vi "get_ValuesByKeyString.vi"(10 "keyString":string, 11 "Json Input":string="{\"code\": 111, \"msg\": \"success\", \"data\": {\"camera_udp_port\": 10001, \"radar_udp_port\": 17000, \"radar_decode_head\": \"AAAA5555\", \"tcp_server_port\": 8888, \"mcu_enable\": 1, \"ntp_enable\": 1, \"radar_get_edition_enable\": 1, \"mcu_get_edition_enable\": 1, \"infer_enable\": 1, \"cpu_min_to_restart_infer\": 20, \"camera_remote_enable\": 1, \"video_save\": 3, \"pronounce_english\": 0, \"zipx_s_service_restart_time_s\": -1, \"http_file_port\": -1, \"max_file_num\": 1000, \"max_file_size\": 2000000000, \"pic_timeSpan_min\": 5, \"mp4_timeSpan_min\": 4, \"pika_rabbitmq_enable\": 0, \"pika_sftp_enable\": 0, \"radar_alarm_score\": 455, \"camera_alarm_score\": 20, \"joint_alarm_score\": 150, \"camera_radar_h_offset_rad\": -0.01, \"confidence_min\": 0.55, \"radarOffset\": 0.0, \"autoMendRadarOffset\": 0, \"autoCalibration\": 0, \"H\": 2.4}}") -> (3 "Values":dbl[](array[numeric]))   [LabVIEW 2022 SP3]
uses:
  <vilib>/Utility/error.llb/Trim Whitespace One-Sided.vi
panel:
  out "Array":string[](array[string])
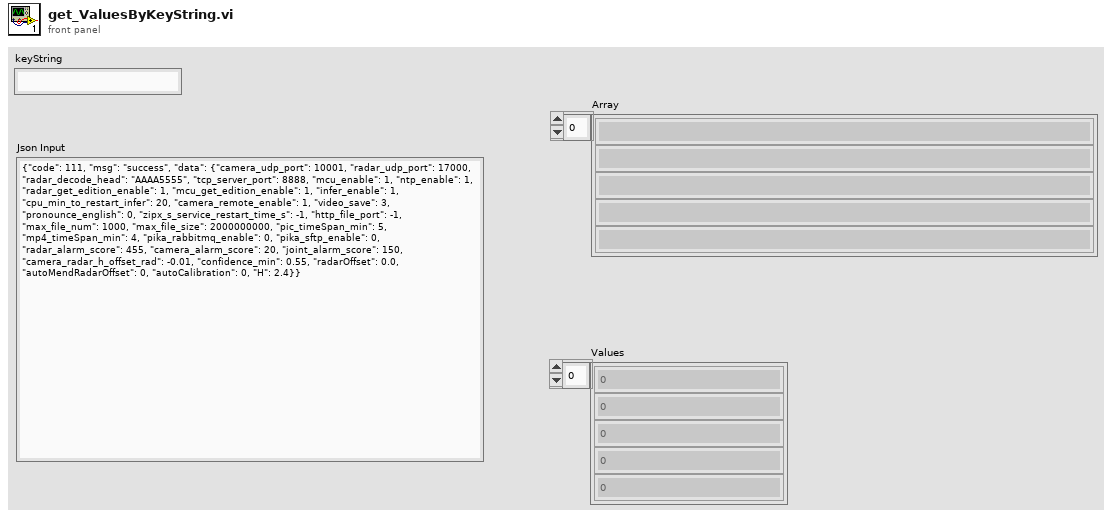
[diagram p1: front panel]
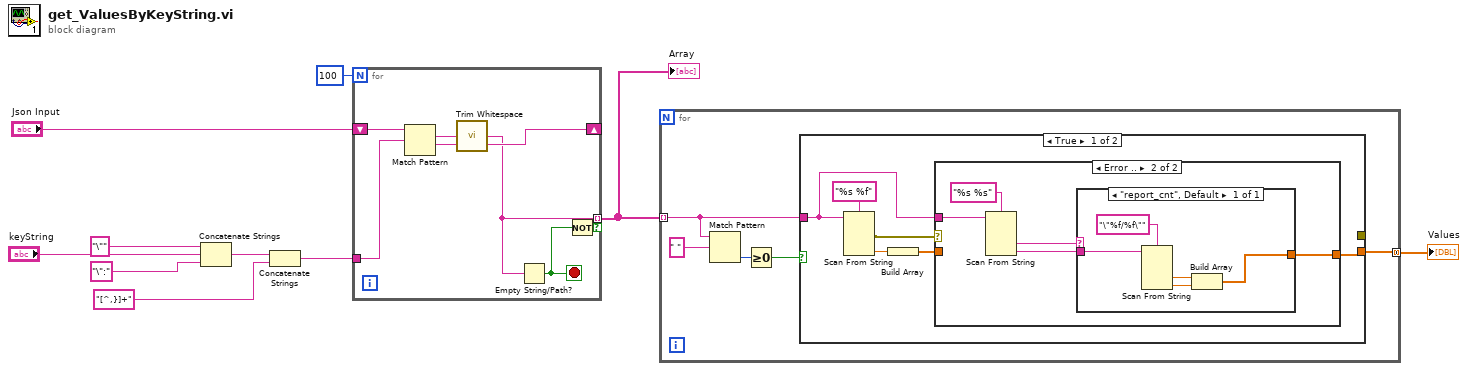
[diagram p0: block diagram]
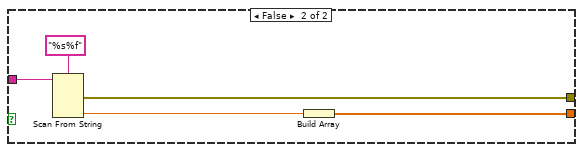
[diagram p3: hidden frame]
diagram:
  n1 = Concatenate Strings("\"" ("string"), "keyString", "\":" ("regular expression")) -> (w6:string)
  n2 = Concatenate Strings(w6, "[^,}]+" ("string")) -> (w5:string)
  n3 = for {
    N: 100 -> [_]
    tunnel: w5 -> [w16]
    shift-right: [w15] -> _
    shift-left: "Json Input" -> [w17]
    tunnel: [w13] -> w2 mode=indexing if=w11
    stop <- w12 stop-if-true
    n4 = Match Pattern(string=w17, regular expression=w16) -> (match substring=w14:string, after substring=w15:string)  [unwired: 1 in, 2 out]
    n5 = call <vilib>:"Trim Whitespace.vi"("string"=w14) -> ("trimmed string"=w13:string)  [unwired: 1 in]
    n6 = Empty String/Path?(string/path=w13) -> (empty?=w12:bool)
    n7 = Not(x=w12) -> (.not. x?=w11:bool)
  }
  "Array" <- w2
  n8 = for {
    tunnel: w2 -> [w21] mode=indexing
    tunnel: [w22] -> w1 mode=concatenating
    n9 = Match Pattern(string=w21, regular expression=" ") -> (offset past match=w19:i32)  [unwired: 1 in, 3 out]
    n10 = Greater Or Equal To 0?(x=w19) -> (x >= 0?=w18:bool)
    n11 = case shown="True" w18 {
      tunnel: [w23 w40] -> w22
      tunnel: w21 -> [w25 w42]
      tunnel: [_ w41] -> _
      frame True {
        n12 = Scan From String(format string="%s %f", input string=w25) -> (error out=w26:errorcluster, output 2=w27:dbl)  [unwired: 5 in, 2 out]
        n13 = Build Array(w27) -> (w24:dbl[])
        n14 = case shown="Error .." w26 {
          tunnel: w25 -> [_ w34]
          tunnel: [w29 w30] -> w23
          tunnel: w24 -> [w29 _]
          frame No Error {
          }
          frame Error {
            n15 = Scan From String(format string="%s %s", input string=w34) -> (output 1=w31:string, output 2=w32:string)  [unwired: 4 in, 3 out]
            n16 = case shown="\"report_cnt\", Default" w31 {
              tunnel: w32 -> [w38]
              tunnel: [w35] -> w30
              frame "report_cnt", Default {
                n17 = Scan From String(format string="\"%f/%f\"", input string=w38) -> (output 1=w37:dbl, output 2=w36:dbl)  [unwired: 4 in, 3 out]
                n18 = Build Array(w37, w36) -> (w35:dbl[])
              }
            }
          }
        }
      }
      frame False {
        n19 = Scan From String(format string="%s%f", input string=w42) -> (error out=w41:errorcluster, output 2=w43:dbl)  [unwired: 5 in, 2 out]
        n20 = Build Array(w43) -> (w40:dbl[])
      }
    }
  }
  "Values" <- w1
